vi "Throw Data Replay Parse Warning.vi"(6 "Controls":string[](array[string]), 7 "Replay":string, 8 "Found Numbers":string[](array[string]), 9 "All numbers same?":bool, 10 "All controls present?":bool, 11 "Found Controls":bool[](array[boolean])) -> ()   [LabVIEW 2011, in "Engine Sim System Explorer.lvlib"]
uses:
  Engine Sim System Explorer.lvlib
  <userlib>/_OpenG.lib/array/array.llb/Conditional Auto-Indexing Tunnel (String)__ogtk.vi
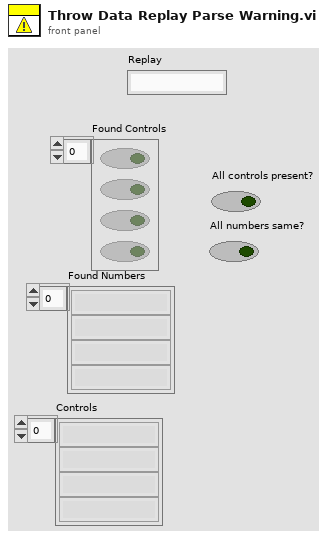
[diagram p1: front panel]
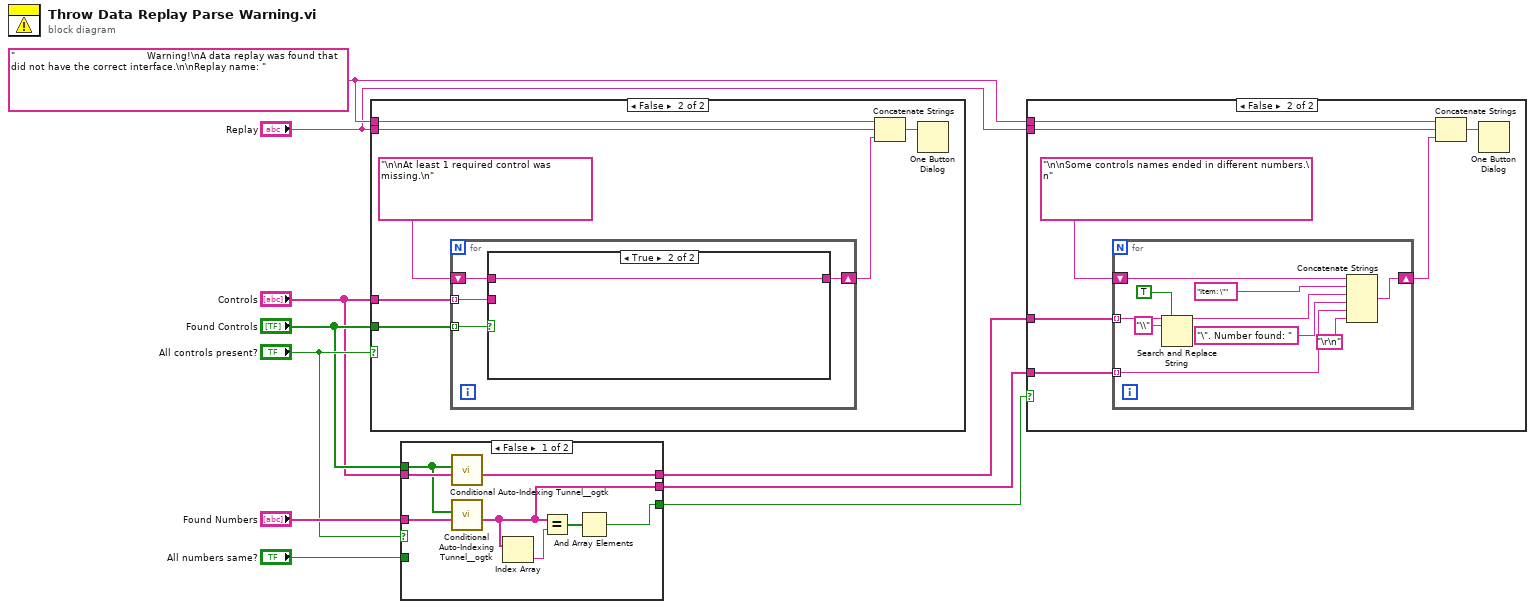
[diagram p0: block diagram]
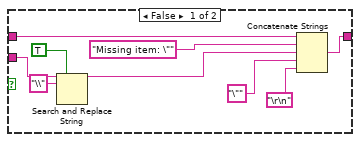
[diagram p5: hidden frame]
diagram:
  w10 = "                                            Warning!\nA data replay was found that did not have the correct interface.\n\nReplay name: " ("message")
  n1 = case shown="False" "All controls present?" {
    tunnel: "Controls" -> [_ w17]
    tunnel: "Found Controls" -> [_ w15]
    tunnel: w10 -> [_ w12]
    tunnel: "Replay" -> [_ w11]
    frame True {
    }
    frame False {
      n2 = for {
        tunnel: w17 -> [w20] mode=indexing
        shift-right: [w19] -> w13
        shift-left: "\n\nAt least 1 required control was missing.\n" -> [w21]
        tunnel: w15 -> [w18] mode=indexing
        n3 = case shown="True" w18 {
          tunnel: w21 -> [w30 w31]
          tunnel: w20 -> [w28 _]
          tunnel: [w23 w31] -> w19
          frame False {
            n4 = Search and Replace String(replace all?=TRUE ("replace all? (F)"), input string=w28, search string="\\") -> (result string=w25:string)  [unwired: 5 in, 3 out]
            n5 = Concatenate Strings(w30, "Missing item: \"", w25, "\"", "\r\n") -> (w23:string)
          }
          frame True {
          }
        }
      }
      n6 = Concatenate Strings(w12, w11, w13) -> (w14:string)
      n7 = One Button Dialog(message=w14) -> ()  [unwired: 1 in, 1 out]
    }
  }
  n8 = case shown="False" "All controls present?" {
    tunnel: "Found Numbers" -> [w39 w40]
    tunnel: [w36 w42] -> w7
    tunnel: "All numbers same?" -> [_ w42]
    tunnel: "Found Controls" -> [w32 _]
    tunnel: "Controls" -> [w35 w41]
    tunnel: [w34 w41] -> w2
    tunnel: [w33 w40] -> w1
    frame False {
      n9 = call-poly <userlib>:"Conditional Auto-Indexing Tunnel__ogtk.vi"("Array in"=w35, "Elements to keep"=w32) -> ("Filtered Array out"=w34:string[])  [unwired: 5 in]
      n10 = call-poly <userlib>:"Conditional Auto-Indexing Tunnel__ogtk.vi"("Array in"=w39, "Elements to keep"=w32) -> ("Filtered Array out"=w33:string[])  [unwired: 5 in]
      n11 = Index Array(array=w33) -> (element=w38:string)  [unwired: 1 in]
      n12 = Equal?(x=w33, y=w38) -> (x = y?=w37:bool[])
      n13 = And Array Elements(Boolean array=w37) -> (logical AND=w36:bool)
    }
    frame True {
    }
  }
  n14 = case shown="False" w7 {
    tunnel: w2 -> [_ w43]
    tunnel: w10 -> [_ w48]
    tunnel: "Replay" -> [_ w47]
    tunnel: w1 -> [_ w45]
    frame True {
    }
    frame False {
      n15 = for {
        tunnel: w43 -> [w57] mode=indexing
        shift-right: [w50] -> w44
        shift-left: "\n\nSome controls names ended in different numbers.\n" -> [w59]
        tunnel: w45 -> [w52] mode=indexing
        n16 = Search and Replace String(replace all?=TRUE ("replace all? (F)"), input string=w57, search string="\\") -> (result string=w54:string)  [unwired: 5 in, 3 out]
        n17 = Concatenate Strings(w59, "Item: \"", w54, "\". Number found: ", w52, "\r\n") -> (w50:string)
      }
      n18 = Concatenate Strings(w48, w47, w44) -> (w49:string)
      n19 = One Button Dialog(message=w49) -> ()  [unwired: 1 in, 1 out]
    }
  }
